vi "SpectrumGraph.vi"() -> ()   [LabVIEW 2014]
uses:
  <vilib>/Utility/file.llb/Read From Spreadsheet File (DBL).vi
  <vilib>/Utility/file.llb/Write To Spreadsheet File (DBL).vi
panel:
  out "appended path":path
  out "Time delay (ms)":u32=608
  in  "Calculate FWHM":bool
  out "after":i32=2048
  out "before":i32=2048
  in  "Reduce Array Size (2^nTimes) 2":i32
  in  "Gaussian FIT\nMax Itterations":u32=5
  out "FWHM [nm]":dbl=4.986064808349851 format="%#_4p"
  out "XY Graph":cluster{dbl[], dbl[]}[](graph)
  in  "Save GIF":bool
  out "XY Graph GIF":cluster{dbl[], dbl[]}(graph)
  out "Energy [J]":dbl=0.00026915 format="%#_6p"
  in  "Save Spectrum":bool
  out "Especs reduced":i32=20
  out "XY Graph":cluster{dbl[], dbl[]}(graph)
  in  "Reduce Array Size (2^nTimes)":i32
  out "Points":i32=2048
  out "Points reduced":i32=2048
  out "Spectrun File out":string
  out "Spectrun File in":string="Andre-Smp-101-Spectrum mar-04-2021 Time 21-10.spt"
  in  "Divider Factor":i32=5
  out "Total Specs":i32=105
  in  "Load Spectrum":bool
  in  "Select Spectrum Graph":dbl(slide)=98.0 min=1.0 max=1000.0 step=1.0 scale=0.9..105.0
  # "Fazer rotina que escolhe larguras da linha dos graficos"
  # "palette de cor das linhas"
  # "opcao de recortar o grafico em lambda"
  # "Analise do Erro em função da densidade de pontos e numero de interações da Gaussiana"
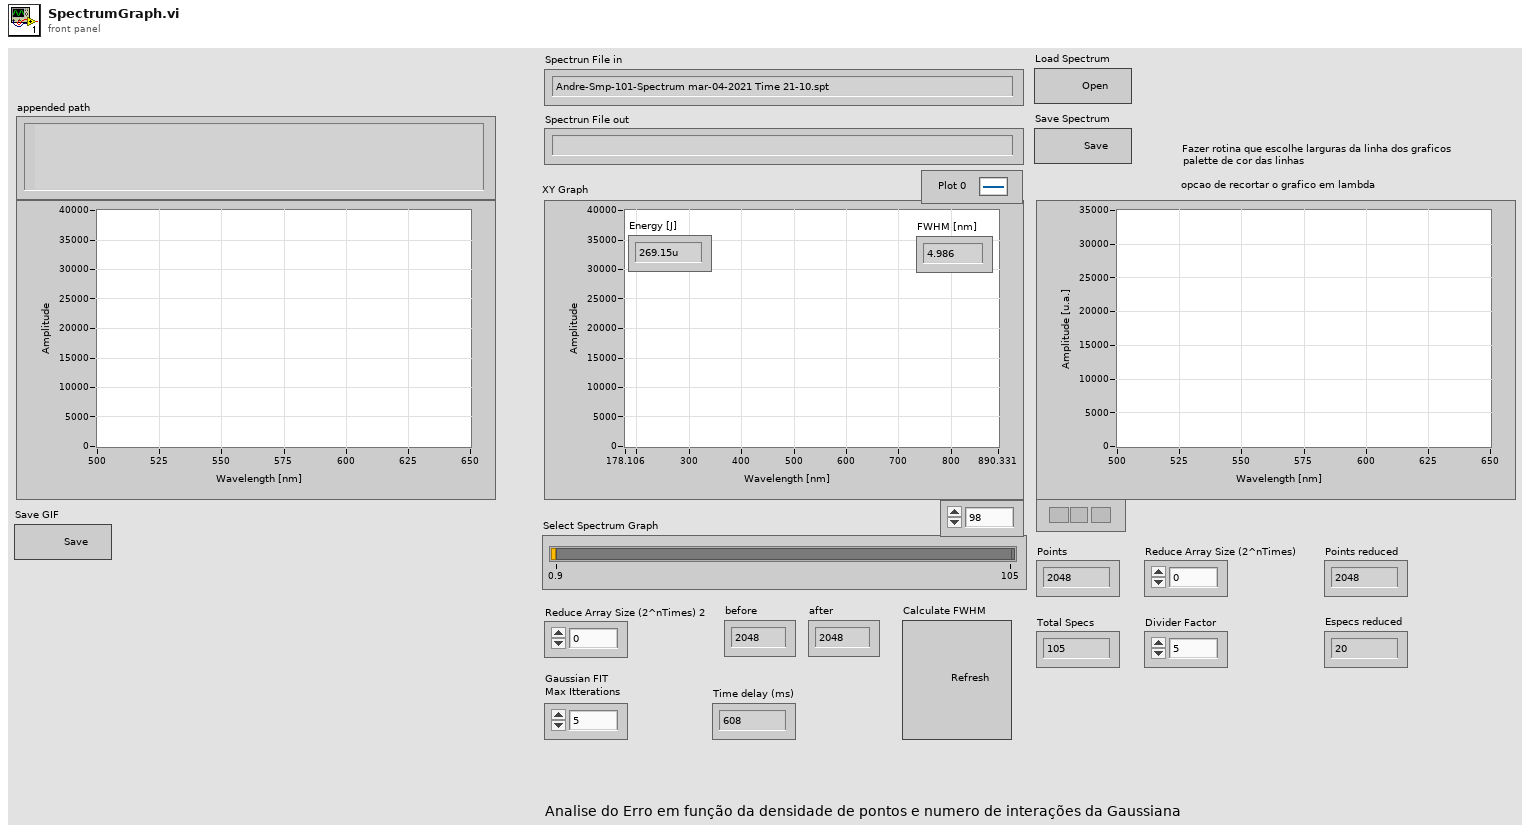
[diagram p1: front panel]
types:
  T1 = enum16{"waitForEvent", "loadFile", "reduceSpecs", "reducePoints", "saveFile", "FWHM", "SaveGIF"}
  T2 = enum16{"waitForEvent", "loadFile", "reduceSpecs", "reducePoints", "saveFile"}
  T3 = enum16{"waitForEvent", "loadFile", "reduceSpecs", "reducePoints", "saveFile", "FWHM"}
  T4 = enum16{"open", "replace", "create", "open or create", "replace or create", "replace or create with confirmation"}
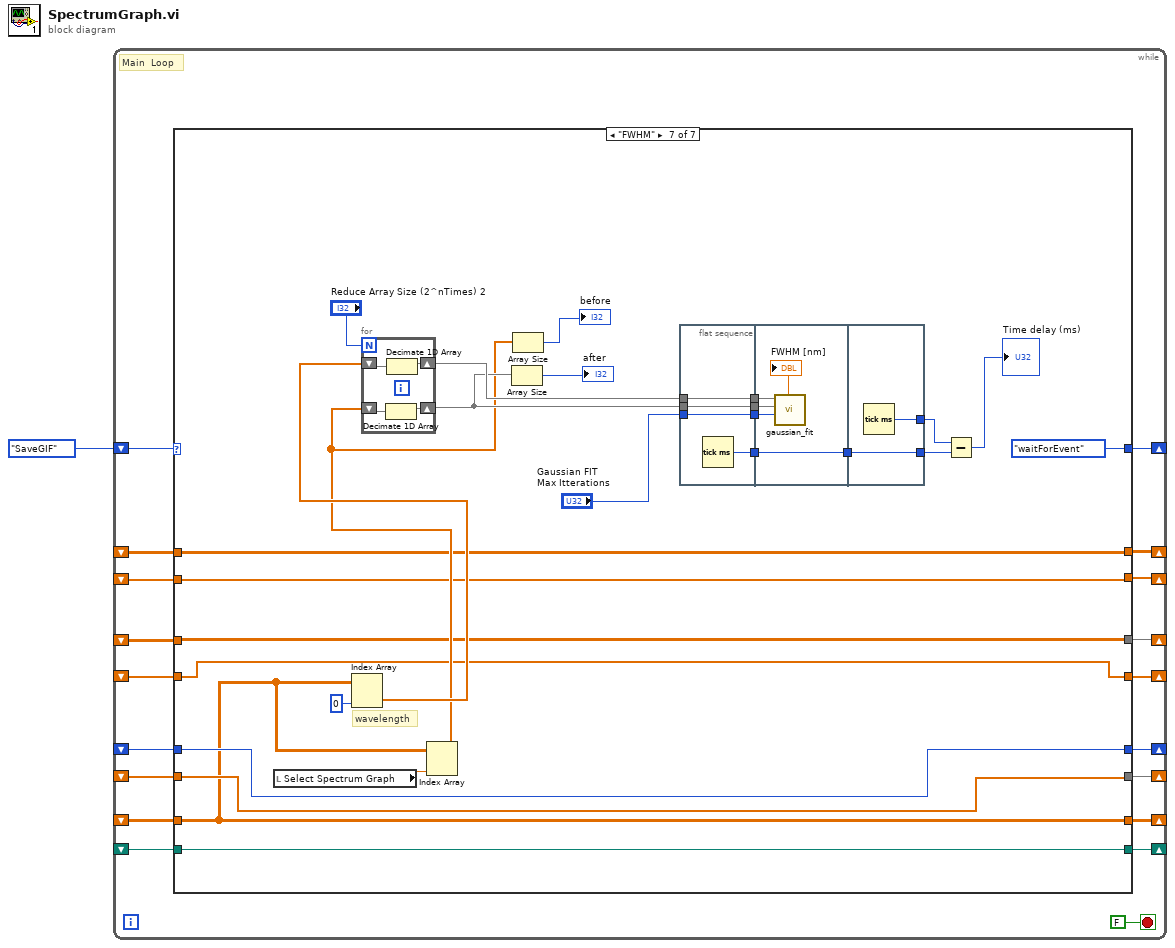
[diagram p0: block diagram]
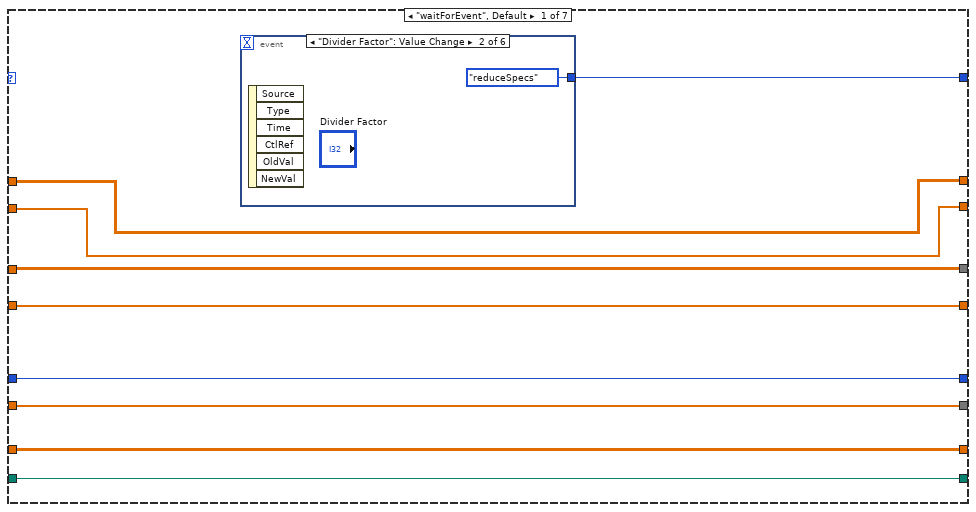
[diagram p2: hidden frame]
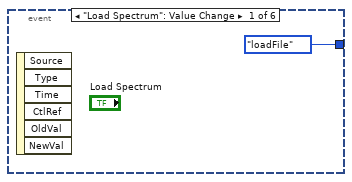
[diagram p3: hidden frame]
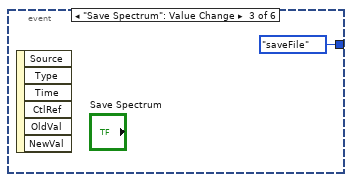
[diagram p4: hidden frame]
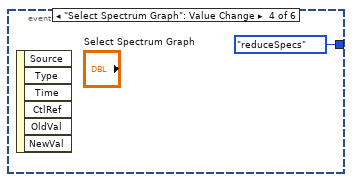
[diagram p5: hidden frame]
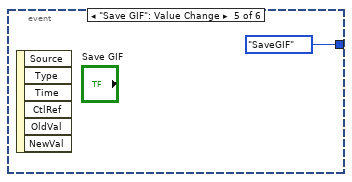
[diagram p6: hidden frame]
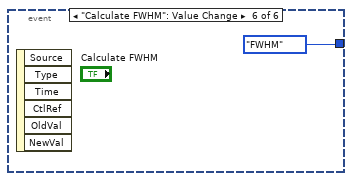
[diagram p7: hidden frame]
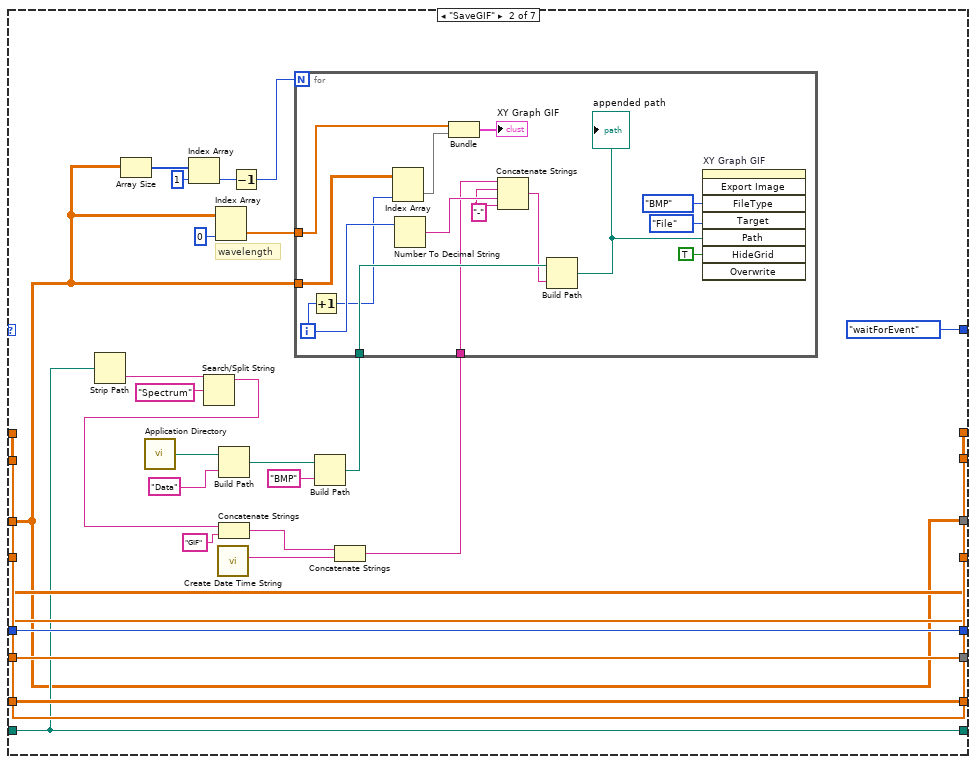
[diagram p8: hidden frame]
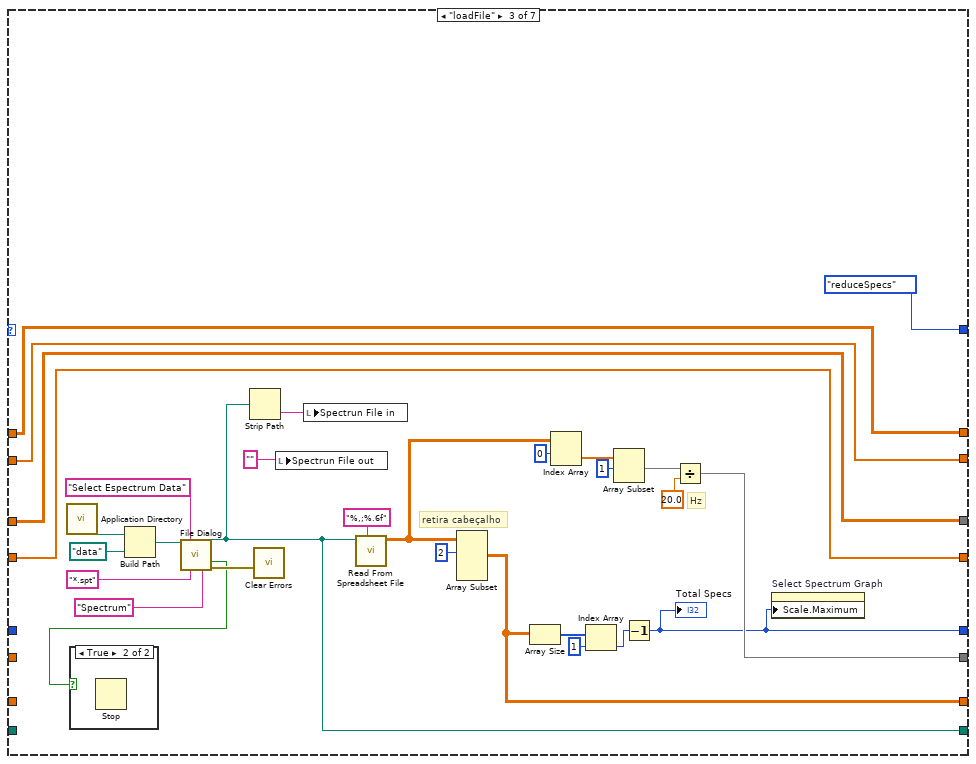
[diagram p9: hidden frame]
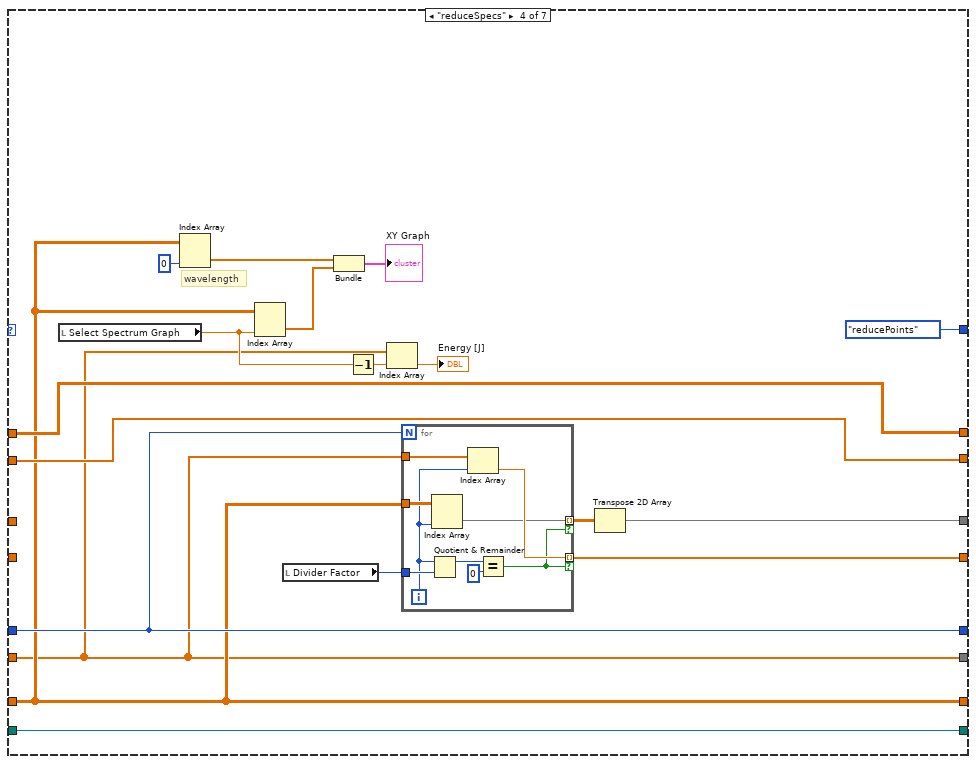
[diagram p11: hidden frame]
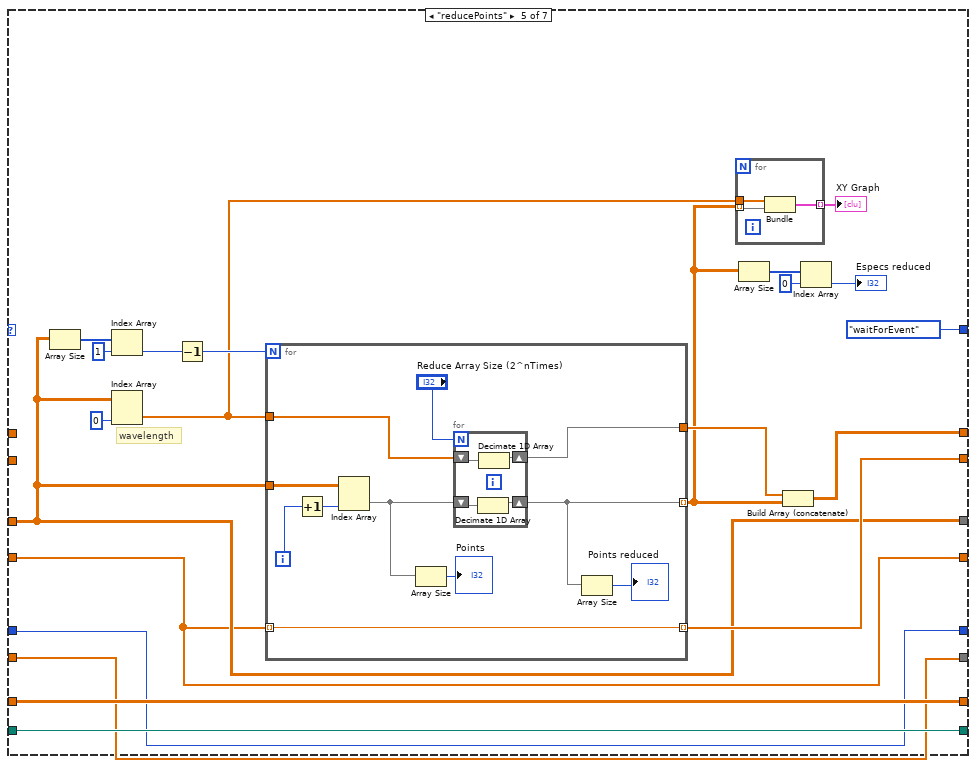
[diagram p12: hidden frame]
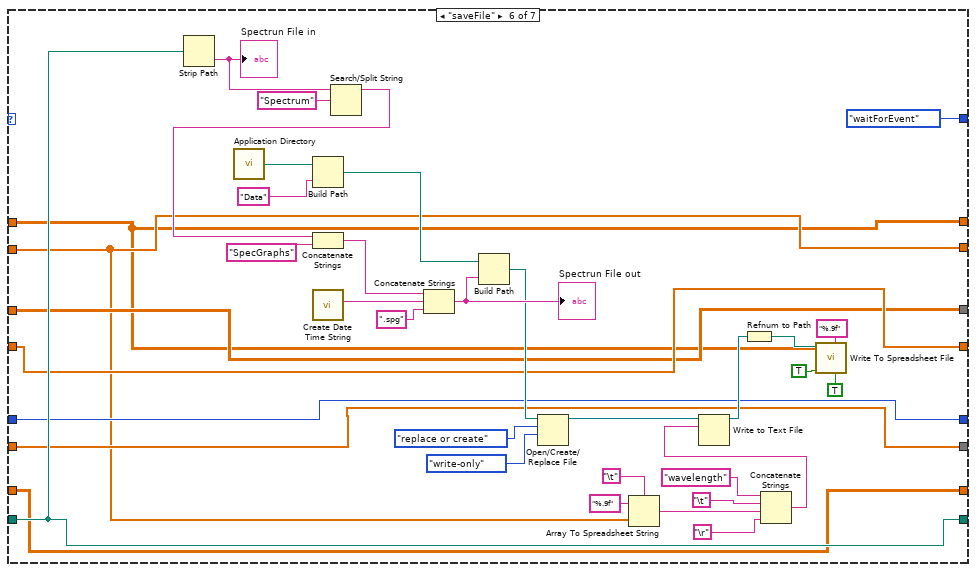
[diagram p13: hidden frame]
diagram:
  n1 = while {
    shift-right: [w18] -> _
    shift-left: T1."SaveGIF" -> [w19]
    shift-right: [w17] -> _
    shift-left: _ -> [w16]
    shift-right: [w15] -> _
    shift-left: _ -> [w14]
    shift-right: [w13] -> _
    shift-left: _ -> [w2]
    shift-right: [w12] -> _
    shift-left: _ -> [w11]
    shift-right: [w10] -> _
    shift-left: _ -> [w9]
    shift-right: [w8] -> _
    shift-left: _ -> [w7]
    shift-right: [w6] -> _
    shift-left: _ -> [w5]
    shift-right: [w4] -> _
    shift-left: _ -> [w3]
    stop <- FALSE stop-if-true
    # "Main  Loop"
    n2 = case shown="\"FWHM\"" w19 {
      tunnel: [w29 T1."waitForEvent" T2."reduceSpecs" T2."reducePoints" T2."waitForEvent" T2."waitForEvent" T2."waitForEvent"] -> w18
      tunnel: [w26 w61 w87 w112 w138 w179 w212] -> w15
      tunnel: [w25 w60 w81 w119 w139 w178 w213] -> w12
      tunnel: [w27 w54 w86 w114 w142 w180 w210] -> w17
      tunnel: [w28 w44 w80 w120 w143 w181 w211] -> w13
      tunnel: w16 -> [w27 w54 _ w114 w142 w180 w210]
      tunnel: w14 -> [w26 w61 _ w112 w138 w179 w212]
      tunnel: w11 -> [w25 w60 _ w119 w139 w178 w213]
      tunnel: [w23 w36 w84 w124 w141 w176 w215] -> w10
      tunnel: w9 -> [w23 w36 w84 _ w141 w176 w215]
      tunnel: [w24 w59 w85 w123 w140 w177 w214] -> w8
      tunnel: w7 -> [w24 w59 w85 _ w140 w177 w214]
      tunnel: [w21 w57 w82 w117 w146 w174 w217] -> w6
      tunnel: w5 -> [w21 w57 w82 w117 _ w174 w217]
      tunnel: [w22 w58 w83 w118 w145 w175 w216] -> w4
      tunnel: w3 -> [w22 w58 w83 w118 _ w175 w216]
      tunnel: w2 -> [w28 w44 _ w120 w143 w181 w211]
      frame "waitForEvent", Default {
        n3 = event shown="[1] \"Divider Factor\": Value Change" {
          selector: _ -> [_ _ _ _ _ _]
          dyn-events: _ -> [_ _ _ _ _ _]
          timeout: _ -> [_ _ _ _ _ _]
          tunnel: [T2."loadFile" T2."reduceSpecs" T2."saveFile" T2."reduceSpecs" T1."SaveGIF" T3."FWHM"] -> w29
          event "Load Spectrum": Value Change {
            n4 = event-data() -> ()  [unwired: 1 in, 6 out]
          }
          event "Divider Factor": Value Change {
            n5 = event-data() -> ()  [unwired: 1 in, 6 out]
          }
          event "Save Spectrum": Value Change {
            n6 = event-data() -> ()  [unwired: 1 in, 6 out]
          }
          event "Select Spectrum Graph": Value Change {
            n7 = event-data() -> ()  [unwired: 1 in, 6 out]
          }
          event "Save GIF": Value Change {
            n8 = event-data() -> ()  [unwired: 1 in, 6 out]
          }
          event "Calculate FWHM": Value Change {
            n9 = event-data() -> ()  [unwired: 1 in, 6 out]
          }
        }
      }
      frame "SaveGIF" {
        # "wavelength"
        n10 = Strip Path(path=w44) -> (name=w49:string)  [unwired: 1 out]
        n11 = Array Size(array=w36) -> (size(s)=w51:i32[])
        n12 = call <vilib>:"Application Directory.vi"() -> ("Application Directory"=w46:path)
        n13 = Index Array(array=w51, index=1) -> (element=w52:i32)
        n14 = Search/Split String(string=w49, search string/char (-)="Spectrum") -> (substring before match=w40:string)  [unwired: 1 in, 2 out]
        n15 = Index Array(array=w36, index (col)=0 ("disabled index (col)")) -> (element=w55:dbl[])  [unwired: 1 in]
        n16 = call "Create Date Time String.vi"() -> ("Date/Time String"=w47:string)  [unwired: 10 in, 1 out]
        n17 = Build Path(base path=w46, name or relative path="Data" ("prompt (Create Folder)")) -> (appended path=w45:path)
        n18 = Concatenate Strings(w40, "GIF" ("string")) -> (w41:string)
        n19 = Decrement(x=w52) -> (x-1=w50:i32)
        n20 = Build Path(base path=w45, name or relative path="BMP") -> (appended path=w38:path)
        n21 = Concatenate Strings(w41, w47) -> (w37:string)
        n22 = for {
          N: w50 -> [_]
          tunnel: w55 -> [w77]
          tunnel: w36 -> [w75]
          tunnel: w38 -> [w70]
          tunnel: w37 -> [w66]
          i -> [w69]
          w67 = "-" ("string")
          n23 = Increment(x=w69) -> (x+1=w63:i32)
          n24 = Index Array(array=w75, index (col)=w63) -> (element=w76:dbl[])  [unwired: 1 in]
          n25 = Number To Decimal String(number=w69) -> (decimal integer string=w68:string)  [unwired: 1 in]
          n26 = Bundle(w77, w76) -> (→"XY Graph GIF":cluster{dbl[], dbl[]})  [unwired: 1 in]
          n27 = Concatenate Strings(w66, w67, w68, w67) -> (w65:string)
          n28 = Build Path(base path=w70, name or relative path=w65) -> (appended path=w64:path)
          "appended path" <- w64
          n29 = invoke on="XY Graph GIF" class="XYGraph (strict)" method="Export Image"("FileType"=enum32{"BMP", "EPS", "EMF", "PICT"}."BMP" ("File Type"), "Target"=enum32{"File", "Clipboard"}."File", "Path"=w64, "HideGrid"=TRUE ("Hide Grid")) -> ()  [unwired: 4 in, 8 out]
        }
      }
      frame "loadFile" {
        # "Hz"
        # "retira cabeçalho"
        n30 = call <vilib>:"Application Directory.vi"() -> ("Application Directory"=w102:path)
        n31 = Build Path(base path=w102, name or relative path=path "data") -> (appended path=w101:path)
        n32 = call "File Dialog"("start path"=w101, "prompt"="Select Espectrum Data", "pattern (all files)"="*.spt", "pattern label"="Spectrum") -> ("selected path"=w80:path, "cancelled"=w99:bool, "error out"=w100:errorcluster)  [unwired: 8 in, 1 out]
        n33 = case shown="True" w99 {
          frame False {
          }
          frame True {
            n34 = Stop() -> ()  [unwired: 1 in]
          }
        }
        n35 = Strip Path(path=w80) -> (name=w79:string)  [unwired: 1 out]
        n36 = call <vilib>:"Clear Errors.vi"("error in (no error)"=w100) -> ()  [unwired: 5 in, 2 out]
        n37 = local write "Spectrun File out"("") -> ()
        n38 = local write "Spectrun File in"(w79) -> ()
        n39 = call-poly <vilib>:"Read From Spreadsheet File.vi"("format (%.3f)"="%,;%.6f", "file path (dialog if empty)"=w80) -> ("all rows"=w96:dbl[][])  [unwired: 5 in, 4 out]
        n40 = Array Subset(array=w96, index (row)=2 ("index")) -> (w86:dbl[][])  [unwired: 3 in]
        n41 = Array Size(array=w86) -> (size(s)=w90:i32[])
        n42 = Index Array(array=w96, index (row)=0) -> (element=w94:dbl[])  [unwired: 1 in]
        n43 = Index Array(array=w90, index=1) -> (element=w88:i32)
        n44 = Array Subset(array=w94, index=1) -> (w91:dbl[])  [unwired: 1 in]
        n45 = Decrement(x=w88) -> (x-1=w81:i32)
        "Total Specs" <- w81
        n46 = Divide(x=w91, y=20.0) -> (x/y=w87:dbl[])
        n47 = property on="Select Spectrum Graph" class="Slide (strict)"("Scale.Maximum"=w81) -> ()  [unwired: 2 in, 2 out]
      }
      frame "reduceSpecs" {
        # "wavelength"
        n48 = local read "Select Spectrum Graph"() -> (w113:dbl)
        n49 = Index Array(array=w114, index (col)=0 ("disabled index (col)")) -> (element=w110:dbl[])  [unwired: 1 in]
        n50 = Index Array(array=w114, index (col)=w113) -> (element=w109:dbl[])  [unwired: 1 in]
        n51 = local read "Divider Factor"() -> (w121:i32)
        n52 = Bundle(w110, w109) -> (→"XY Graph":cluster{dbl[], dbl[]})  [unwired: 1 in]
        n53 = Decrement(x=w113) -> (x-1=w108:dbl)
        n54 = Index Array(array=w112, index=w108) -> (element=→"Energy [J]":dbl)
        n55 = for {
          N: w119 -> [_]
          tunnel: w114 -> [w131]
          tunnel: w121 -> [w134]
          tunnel: w112 -> [w130]
          tunnel: [w128] -> w123 mode=indexing if=w126
          tunnel: [w127] -> w125 mode=indexing if=w126
          i -> [w129]
          n56 = Quotient & Remainder(x=w129, y=w134) -> (x-y*floor(x/y)=w133:i32)  [unwired: 1 out]
          n57 = Index Array(array=w131, index (col)=w129) -> (element=w127:dbl[])  [unwired: 1 in]
          n58 = Index Array(array=w130, index=w129) -> (element=w128:dbl)
          n59 = Equal?(x=w133, y=0) -> (x = y?=w126:bool)
        }
        n60 = Transpose 2D Array(2D array=w125) -> (transposed array=w124:dbl[][])
      }
      frame "reducePoints" {
        # "wavelength"
        n61 = Array Size(array=w141) -> (size(s)=w154:i32[])
        n62 = Index Array(array=w154, index=1) -> (element=w151:i32)
        n63 = Index Array(array=w141, index (col)=0 ("disabled index (col)")) -> (element=w136:dbl[])  [unwired: 1 in]
        n64 = Decrement(x=w151) -> (x-1=w150:i32)
        n65 = for {
          N: w150 -> [_]
          tunnel: w141 -> [w169]
          tunnel: w136 -> [w166]
          tunnel: [w162] -> w149
          tunnel: [w161] -> w137 mode=indexing
          tunnel: w140 -> [w159] mode=indexing
          tunnel: [w159] -> w145 mode=indexing
          i -> [w160]
          n66 = Increment(x=w160) -> (x+1=w168:i32)
          n67 = Index Array(array=w169, index (col)=w168) -> (element=w165:dbl[])  [unwired: 1 in]
          n68 = Array Size(array=w165) -> (size(s)=→"Points":i32)
          n69 = for {
            N: "Reduce Array Size (2^nTimes)" -> [_]
            shift-right: [w171] -> w162
            shift-left: w166 -> [w173]
            shift-right: [w170] -> w161
            shift-left: w165 -> [w172]
            n70 = Decimate 1D Array(w172) -> (w170:dbl[])  [unwired: 1 out]
            n71 = Decimate 1D Array(w173) -> (w171:dbl[])  [unwired: 1 out]
          }
          n72 = Array Size(array=w161) -> (size(s)=→"Points reduced":i32)
        }
        n73 = for {
          tunnel: w137 -> [w158] mode=indexing
          tunnel: w136 -> [w157]
          tunnel: [w156] -> w135 mode=indexing
          n74 = Bundle(w157, w158) -> (w156:cluster{dbl[], dbl[]})  [unwired: 1 in]
        }
        "XY Graph" <- w135
        n75 = Array Size(array=w137) -> (size(s)=w152:i32[])
        n76 = Build Array (concatenate)(w149, w137) -> (w146:dbl[][])
        n77 = Index Array(array=w152, index=0) -> (element=→"Especs reduced":i32)
      }
      frame "saveFile" {
        n78 = Strip Path(path=w181) -> (name=w209:string)  [unwired: 1 out]
        "Spectrun File in" <- w209
        n79 = call <vilib>:"Application Directory.vi"() -> ("Application Directory"=w201:path)
        n80 = Build Path(base path=w201, name or relative path="Data" ("prompt (Create Folder)")) -> (appended path=w200:path)
        n81 = call "Create Date Time String.vi"() -> ("Date/Time String"=w207:string)  [unwired: 10 in, 1 out]
        n82 = Search/Split String(string=w209, search string/char (-)="Spectrum") -> (substring before match=w199:string)  [unwired: 1 in, 2 out]
        n83 = Concatenate Strings(w199, "SpecGraphs" ("string")) -> (w203:string)
        n84 = Concatenate Strings(w203, w207, ".spg" ("string")) -> (w205:string)
        "Spectrun File out" <- w205
        n85 = Build Path(base path=w200, name or relative path=w205) -> (appended path=w184:path)
        n86 = Open/Create/Replace File(file path (use dialog)=w184, operation (0:open)=T4."replace or create", access (0:read/write)=enum16{"read/write", "read-only", "write-only"}."write-only") -> (refnum out=w194:refnum<file>)  [unwired: 3 in, 2 out]
        n87 = Array To Spreadsheet String(delimiter (Tab)="\t", array=w175, 3:"%.9f" ("format string")) -> (spreadsheet string=w189:string)
        n88 = Concatenate Strings("wavelength" ("string"), "\t", w189, "\r") -> (w188:string)
        n89 = Write to Text File(file (use dialog)=w194, text=w188) -> (refnum out=w193:refnum<file>)  [unwired: 2 in, 2 out]
        n90 = Refnum to Path(1:w193) -> (0:w198:path)
        n91 = call-poly <vilib>:"Write To Spreadsheet File.vi"("transpose? (no:F)"=TRUE, "format (%.3f)"="%.9f" ("format string"), "append to file? (new file:F)"=TRUE, "2D data"=w174, "file path (dialog if empty)"=w198) -> ()  [unwired: 3 in, 1 out]
      }
      frame "FWHM" {
        # "wavelength"
        n92 = local read "Select Spectrum Graph"() -> (w236:dbl)
        n93 = Index Array(array=w210, index (col)=0 ("disabled index (col)")) -> (element=w219:dbl[])  [unwired: 1 in]
        n94 = Index Array(array=w210, index (col)=w236) -> (element=w218:dbl[])  [unwired: 1 in]
        n95 = for {
          N: "Reduce Array Size (2^nTimes) 2" -> [_]
          shift-right: [w249] -> w230
          shift-left: w219 -> [w251]
          shift-right: [w248] -> w229
          shift-left: w218 -> [w250]
          n96 = Decimate 1D Array(w250) -> (w248:dbl[])  [unwired: 1 out]
          n97 = Decimate 1D Array(w251) -> (w249:dbl[])  [unwired: 1 out]
        }
        n98 = Array Size(array=w229) -> (size(s)=→"after":i32)
        n99 = Array Size(array=w218) -> (size(s)=→"before":i32)
        n100 = flat-sequence {
          tunnel: w229 -> [w238]
          tunnel: w230 -> [w239]
          tunnel: "Gaussian FIT\nMax Itterations" -> [w240]
          tunnel: [w240] -> w228
          tunnel: [w239] -> w227
          tunnel: [w238] -> w226
          tunnel: [w237] -> w223
          tunnel: w228 -> [w245]
          tunnel: w227 -> [w243]
          tunnel: w226 -> [w242]
          tunnel: w223 -> [w241]
          tunnel: [w241] -> w222
          tunnel: [w247] -> w224
          tunnel: w222 -> [w246]
          tunnel: [w246] -> w221
          frame #0 {
            n101 = Tick Count (ms)() -> (millisecond timer value=w237:u32)
          }
          frame #1 {
            n102 = call "gaussian_fit.vi"("Max Itterations"=w245, "Y Values"=w242, "X Values"=w243) -> ("FWHM"=→"FWHM [nm]":dbl)  [unwired: 1 in, 5 out]
          }
          frame #2 {
            n103 = Tick Count (ms)() -> (millisecond timer value=w247:u32)
          }
        }
        n104 = Subtract(x=w224, y=w221) -> (x-y=→"Time delay (ms)":u32)
      }
    }
  }
